vi "DB Delect data(index).vi"(6 "Condtion":string, 7 "code":string, 8 "error in (no error)":errorcluster caption="错误输入（无错误）", 9 "index":i32, 10 "table":string, 11 "Connncet State":T1) -> (0 "error out":errorcluster caption="错误输出", 2 "Boolean":bool, 3 "Connncet State out":T1)   [LabVIEW 2014]
uses:
  <vilib>/addons/database/NI_Database_API.lvlib
  Ctr/Constr.ctl
  <vilib>/addons/database/Connection.llb/Conn ObjectReference.ctl
  Ctr/Conneect State.ctl
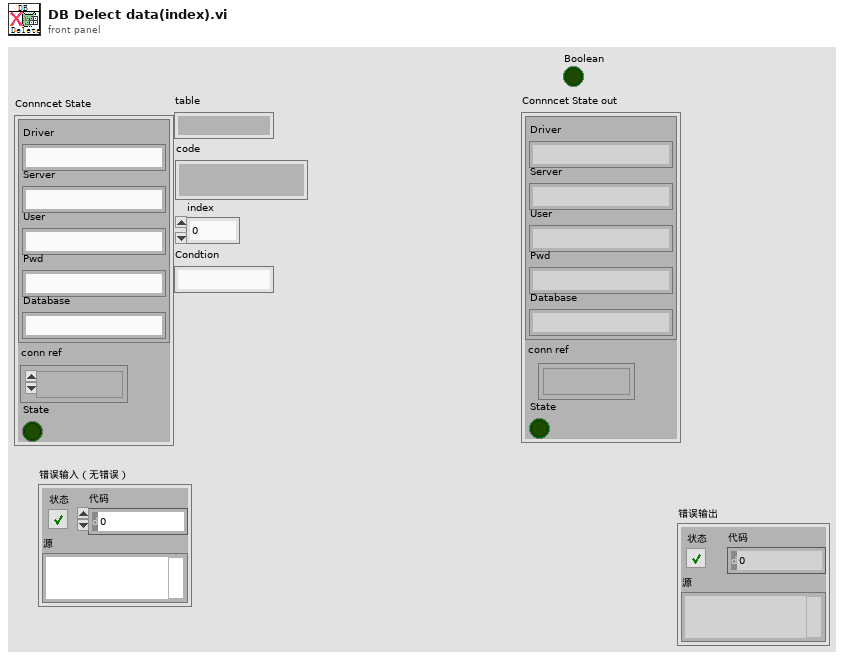
[diagram p1: front panel]
types:
  T1 = typedef "Conneect State.ctl" = cluster{"Constr":T2, "conn ref":T3, "State":bool}
  T2 = typedef "Constr.ctl" = cluster{"Driver":string, "Server":string, "User":string, "Pwd":string, "Database":string}
  T3 = typedef "NI_Database_API.lvlib/Conn ObjectReference.ctl" = refnum<k1>
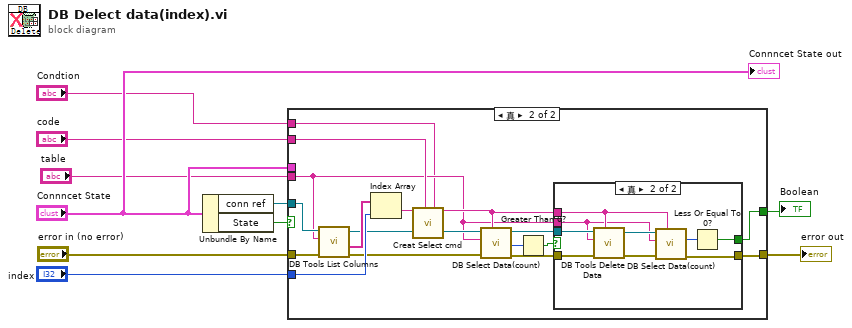
[diagram p0: block diagram]
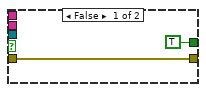
[diagram p3: hidden frame]
diagram:
  n1 = Unbundle By Name("Connncet State") -> ("conn ref"=w3:T3, "State"=w4:bool)
  n2 = case shown="真" w4 {
    tunnel: "error in (no error)" -> [w11 w28]
    tunnel: w3 -> [_ w27]
    tunnel: "table" -> [_ w14]
    tunnel: "code" -> [_ w26]
    tunnel: "Connncet State" -> [_ _]
    tunnel: [w11 w16] -> w6
    tunnel: "index" -> [_ w23]
    tunnel: "Condtion" -> [_ w13]
    tunnel: [_ w12] -> w1
    frame False {
    }
    frame True {
      n3 = call <vilib>:"DB Tools List Columns.vi"("error in (no error)"=w28, "table"=w14, "connection reference"=w27) -> ("error out"=w22:errorcluster, "columns"=w24:string[], "connection reference out"=w21:T3)  [unwired: 1 in, 1 out]
      n4 = Index Array(array=w24, index=w23) -> (element=w25:string)
      n5 = call "Creat Select cmd.vi"("Col"=w25, "Code"=w26, "Condtion"=w13) -> ("Str"=w15:string)  [unwired: 11 in, 1 out]
      n6 = call "DB Select Data(count).vi"("condition"=w15, "error in (no error)"=w22, "table"=w14, "connection reference"=w21) -> ("error out"=w18:errorcluster, "Count"=w20:i32, "connection reference out"=w17:T3)  [unwired: 5 in]
      n7 = Greater Than 0?(x=w20) -> (x > 0?=w19:bool)
      n8 = case shown="真" w19 {
        tunnel: w18 -> [w30 w39]
        tunnel: w17 -> [_ w38]
        tunnel: [w30 w36] -> w16
        tunnel: w15 -> [_ w35]
        tunnel: w14 -> [_ w33]
        tunnel: [TRUE w31] -> w12
        frame False {
        }
        frame True {
          n9 = call <vilib>:"DB Tools Delete Data.vi"("condition"=w35, "error in (no error)"=w39, "table"=w33, "connection reference"=w38) -> ("error out"=w37:errorcluster, "connection reference out"=w34:T3)  [unwired: 6 in]
          n10 = call "DB Select Data(count).vi"("condition"=w35, "error in (no error)"=w37, "table"=w33, "connection reference"=w34) -> ("error out"=w36:errorcluster, "Count"=w32:i32)  [unwired: 5 in, 1 out]
          n11 = Less Or Equal To 0?(x=w32) -> (x <= 0?=w31:bool)
        }
      }
    }
  }
  "error out" <- w6
  "Boolean" <- w1
  "Connncet State out" <- "Connncet State"
